vi "Create (Type Code).vi"(8 "error in":errorcluster, 10 "type code":T1=enum."AnyA", 11 "Value in":refnum<class "Value.lvclass">) -> (0 "error out":errorcluster, 3 "Value out":refnum<class "Value.lvclass">)   [LabVIEW 2020, in "Value.lvlib" / "Value.lvclass"]
uses:
  Value.lvclass
  Type Code.ctl
  Value.lvclass/Value.ctl
  Value.lvlib
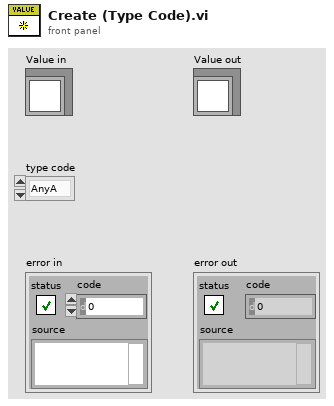
[diagram p1: front panel]
types:
  T1 = typedef "Value.lvlib/Type Code.ctl" = enum8{"Null", "Bool", "BoolA", "Int8", "Int8A", "Int16", "Int16A", "Int32", "Int32A", "Int64", "Int64A", "UInt8", "UInt8A", "UInt16", "UInt16A", "UInt32", "UInt32A", "UInt64", "UInt64A", "Float32", "Float32A", "Float64", "Float64A", "String", "StringA", "Struct", "StructA", "Union", "UnionA", "Any", "AnyA"}
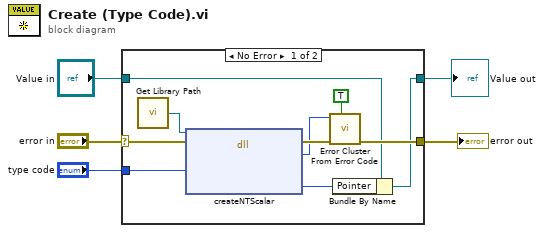
[diagram p0: block diagram]
diagram:
  n1 = case shown="No Error" "error in" {
    selector: "error in" -> [w15 w17]
    tunnel: [w11 w17] -> w5
    tunnel: "type code" -> [w10 _]
    tunnel: "Value in" -> [w7 w16]
    tunnel: [w6 w16] -> w1
    frame No Error {
      n2 = call "Get Library Path.vi"() -> ("Path"=w9:path)  [unwired: 1 in]
      n3 = dll-call lib="?" fn="createNTScalar"(path in=w9, error in=w15, "type_code"=w10) -> (error out=w13:errorcluster, "err_code"=w12:i32, "value"=w8:i64)  [unwired: 3 in, 1 out]
      n4 = call <vilib>:"Error Cluster From Error Code.vi"("show call chain? (False)"=TRUE, "error in (no error)"=w13, "error code (0)"=w12) -> ("error out"=w11:errorcluster)  [unwired: 6 in]
      n5 = Bundle By Name(cluster=w7, "Pointer"=w8) -> (w6:refnum<class "Value.lvclass">)
    }
    frame Error {
    }
  }
  "error out" <- w5
  "Value out" <- w1
